vi "ccd_handle.vi"() -> ()   [LabVIEW 2018]
uses:
  <vilib>/vision/driver/NI_Vision_Acquisition_Software.lvlib
  <vilib>/userdefined/High Color/IMAQdx.ctl
  <vilib>/vision/Image Controls.llb/IMAQ Image.ctl
panel:
  in  "输出簇 2":T2
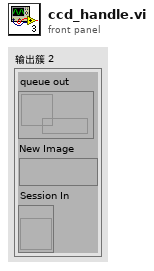
[diagram p1: front panel]
types:
  T1 = typedef "IMAQ Image.ctl" = refnum<image>
  T2 = cluster{"queue out":refnum<queue>, "New Image":T1, "Session In":refnum<vi>}
  T3 = typedef "IMAQdx.ctl" = refnum<k21>
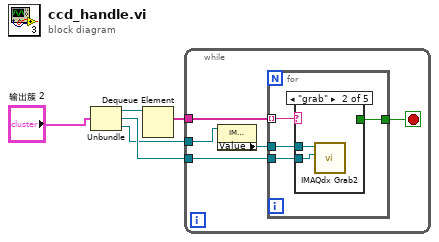
[diagram p0: block diagram]
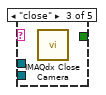
[diagram p3: hidden frame]
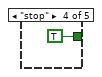
[diagram p4: hidden frame]
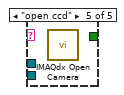
[diagram p5: hidden frame]
diagram:
  n1 = Unbundle("输出簇 2") -> ("queue out"=w4:refnum<queue>, "New Image"=w3:T1, "Session In"=w2:refnum<vi>)
  n2 = Dequeue Element(queue=w4) -> (element=w5:string[])  [unwired: 2 in, 3 out]
  n3 = while {
    tunnel: w5 -> [w10]
    tunnel: w2 -> [w7]
    tunnel: w3 -> [w9]
    stop <- w8 stop-if-true
    n4 = property class="IMAQdx (严格)"(reference=w7) -> ("Value"=w6:T3)  [unwired: 1 in, 2 out]
    n5 = for {
      tunnel: w10 -> [w14] mode=indexing
      tunnel: w9 -> [w13]
      tunnel: [w12] -> w8
      tunnel: w6 -> [w11]
      n6 = case shown="\"grab\"" w14 {
        tunnel: w13 -> [_ w16 _ _ _]
        tunnel: [_ _ _ TRUE _] -> w12
        tunnel: w11 -> [_ w15 _ _ _]
        frame "con ccd" {
        }
        frame "grab" {
          n7 = call <vilib>:"IMAQdx Grab2.vi"("Image In"=w16, "Session In"=w15) -> ()  [unwired: 6 in, 4 out]
        }
        frame "close" {
          n8 = call <vilib>:"IMAQdx Close Camera.vi"() -> ()  [unwired: 11 in, 1 out]
        }
        frame "stop" {
        }
        frame "open ccd" {
          n9 = call <vilib>:"IMAQdx Open Camera.vi"() -> ()  [unwired: 10 in, 2 out]
        }
      }
    }
  }
